vi "GeTextValue.vi"(7 "index":i32, 9 "Area":i32, 11 "ArrayTxt":string[](array[string])) -> (0 "Y+H":i32, 1 "X+W":i32, 2 "Y":i32, 3 "X":i32, 4 "FullText":string)   [LabVIEW 2018]
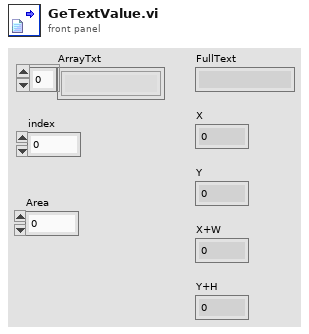
[diagram p1: front panel]
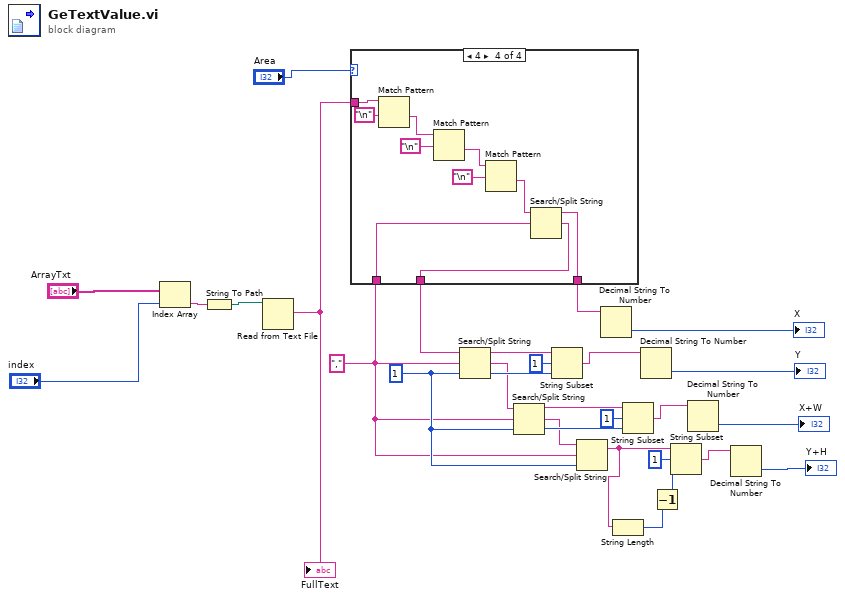
[diagram p0: block diagram]
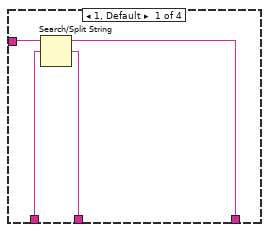
[diagram p2: hidden frame]
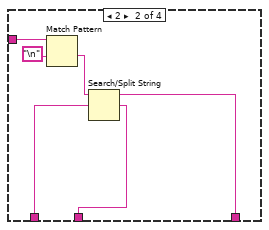
[diagram p3: hidden frame]
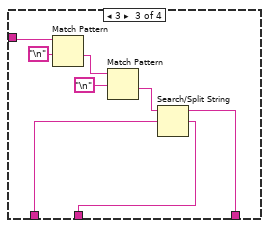
[diagram p4: hidden frame]
diagram:
  w15 = 1 ("offset (0)")
  w7 = "," ("search string/char (-)")
  n1 = Index Array(array="ArrayTxt", index="index") -> (element=w11:string)
  n2 = String To Path(string=w11) -> (path=w12:path)
  n3 = Read from Text File(file (use dialog)=w12) -> (text=w4:string)  [unwired: 3 in, 3 out]
  "FullText" <- w4
  n4 = case shown="4" "Area" {
    tunnel: w4 -> [w33 w38 w45 w53]
    tunnel: w7 -> [w32 w36 w42 w50]
    tunnel: [w31 w34 w40 w48] -> w5
    tunnel: [w30 w35 w41 w49] -> w6
    frame 1, Default {
      n5 = Search/Split String(string=w33, search string/char (-)=w32) -> (substring before match=w31:string, match + rest of string=w30:string)  [unwired: 1 in, 1 out]
    }
    frame 2 {
      n6 = Match Pattern(string=w38, regular expression="\n") -> (after substring=w37:string)  [unwired: 1 in, 3 out]
      n7 = Search/Split String(string=w37, search string/char (-)=w36) -> (substring before match=w34:string, match + rest of string=w35:string)  [unwired: 1 in, 1 out]
    }
    frame 3 {
      n8 = Match Pattern(string=w45, regular expression="\n") -> (after substring=w44:string)  [unwired: 1 in, 3 out]
      n9 = Match Pattern(string=w44, regular expression="\n") -> (after substring=w43:string)  [unwired: 1 in, 3 out]
      n10 = Search/Split String(string=w43, search string/char (-)=w42) -> (substring before match=w40:string, match + rest of string=w41:string)  [unwired: 1 in, 1 out]
    }
    frame 4 {
      n11 = Match Pattern(string=w53, regular expression="\n") -> (after substring=w57:string)  [unwired: 1 in, 3 out]
      n12 = Match Pattern(string=w57, regular expression="\n") -> (after substring=w52:string)  [unwired: 1 in, 3 out]
      n13 = Match Pattern(string=w52, regular expression="\n") -> (after substring=w51:string)  [unwired: 1 in, 3 out]
      n14 = Search/Split String(string=w51, search string/char (-)=w50) -> (substring before match=w48:string, match + rest of string=w49:string)  [unwired: 1 in, 1 out]
    }
  }
  n15 = Search/Split String(string=w6, search string/char (-)=w7, offset (0)=w15) -> (substring before match=w16:string, match + rest of string=w13:string, offset of match=w17:i32)
  n16 = Search/Split String(string=w13, search string/char (-)=w7, offset (0)=w15) -> (substring before match=w21:string, match + rest of string=w14:string, offset of match=w22:i32)
  n17 = String Subset(string=w16, offset (0)=1, length (rest)=w17) -> (substring=w23:string)
  n18 = Search/Split String(string=w14, search string/char (-)=w7, offset (0)=w15) -> (substring before match=w3:string)  [unwired: 2 out]
  n19 = Decimal String To Number(string=w5) -> (number=→"X":i32)  [unwired: 2 in, 1 out]
  n20 = String Length(string=w3) -> (length=w2:i32)
  n21 = String Subset(string=w21, offset (0)=1, length (rest)=w22) -> (substring=w24:string)
  n22 = Decimal String To Number(string=w23) -> (number=→"Y":i32)  [unwired: 2 in, 1 out]
  n23 = Decrement(x=w2) -> (x-1=w1:i32)
  n24 = String Subset(string=w3, offset (0)=1, length (rest)=w1) -> (substring=w25:string)
  n25 = Decimal String To Number(string=w24) -> (number=→"X+W":i32)  [unwired: 2 in, 1 out]
  n26 = Decimal String To Number(string=w25) -> (number=→"Y+H":i32)  [unwired: 2 in, 1 out]
